vi "Verify File.vi"(8 "error in (no error)":errorcluster, 9 "where in bucket to search (prefix)":string, 10 "file to check":path, 11 "Data.S3":refnum<class "Data.S3.lvclass">) -> (0 "error out":errorcluster, 2 "found somewhere in prefix":bool, 3 "Data.S3 out":refnum<class "Data.S3.lvclass">)   [LabVIEW 2020, in "Data.S3.lvclass"]
uses:
  Data.S3.lvclass
  <vilib>/AWS Toolkit/S3/Object Content.ctl
  <vilib>/AWS Toolkit/S3/Storage Class.ctl
  <vilib>/AWS Toolkit/S3/Owner.ctl
  Data.S3.lvclass/Data.S3.ctl
  <vilib>/AWS Toolkit/S3/Bucket/Bucket.lvclass
  <vilib>/AWS Toolkit/S3/NI_AWS_S3.lvlib
panel:
  out "Objects":T1[](array[typedef])
  # "<- can be just file name or path including file\n***doesn't find files with apostrophes in them\nand probably other characters"
  # "prefix to search\ni.e. 'PPMS2' to search within PPMS2\nor 'PPMS2/SA' to search for things\nstarting with SA in PPMS2 folder"
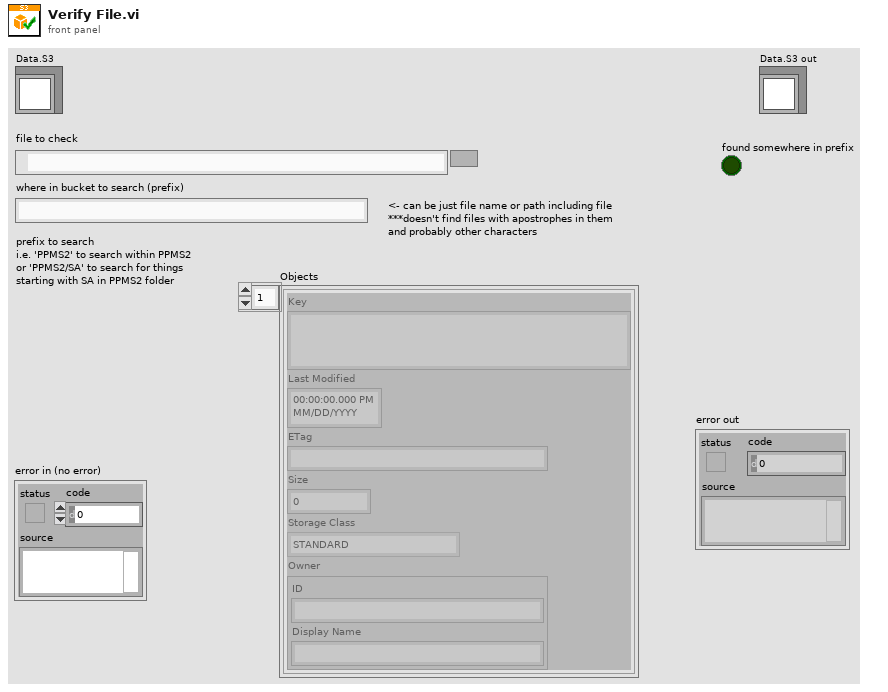
[diagram p1: front panel]
types:
  T1 = typedef "NI_AWS_S3.lvlib/Object Content.ctl" = cluster{"Key":string, "Last Modified":timestamp, "ETag":string, "Size":u64, "Storage Class":T2, "Owner":T3}
  T2 = typedef "NI_AWS_S3.lvlib/Storage Class.ctl" = enum16{"STANDARD", "REDUCED_REDUNDANCY"}
  T3 = typedef "NI_AWS_S3.lvlib/Owner.ctl" = cluster{"ID":string, "Display Name":string}
  T4 = typedef "NI_AWS_Core.lvlib/HTTP Request.lvclass/AWS Credentials.ctl" = cluster{"Access Key":string, "Secret Key":string}
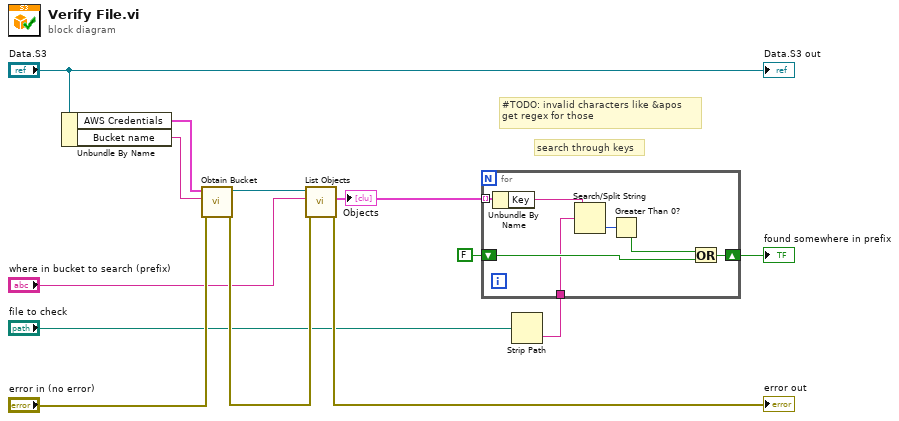
[diagram p0: block diagram]
diagram:
  # "search through keys"
  # "#TODO: invalid characters like &apos\nget regex for those"
  n1 = Unbundle By Name("Data.S3") -> ("AWS Credentials"=w3:T4, "Bucket name"=w2:string)
  n2 = call <vilib>:"Obtain Bucket.vi"("error in (no error)"="error in (no error)", "Bucket name"=w2, "AWS Credentials"=w3) -> ("error out"=w11:errorcluster, "Bucket"=w12:refnum<class "Bucket.lvclass">)  [unwired: 7 in]
  n3 = call <vilib>:"List Objects.vi"("error in (no error)"=w11, "Prefix"="where in bucket to search (prefix)", "Bucket in"=w12) -> ("error out"=→"error out":errorcluster, "Objects"=w8:T1[])  [unwired: 5 in, 2 out]
  "Objects" <- w8
  n4 = Strip Path(path="file to check") -> (name=w7:string)  [unwired: 1 out]
  n5 = for {
    tunnel: w8 -> [w20] mode=indexing
    tunnel: w7 -> [w16]
    shift-right: [w19] -> w6
    shift-left: FALSE -> [w18]
    n6 = Unbundle By Name(w20) -> ("Key"=w17:string)
    n7 = Search/Split String(string=w17, search string/char (-)=w16) -> (offset of match=w15:i32)  [unwired: 1 in, 2 out]
    n8 = Greater Than 0?(x=w15) -> (x > 0?=w14:bool)
    n9 = Or(x=w14, y=w18) -> (x .or. y?=w19:bool)
  }
  "found somewhere in prefix" <- w6
  "Data.S3 out" <- "Data.S3"
